vi "Save image to Tiff stack file.vi"(6 "error in":errorcluster, 8 "Tiff string\n (unsigned byte array)":u8[](array[numeric]), 9 "Path":path) -> (0 "error out":errorcluster)   [LabVIEW 2013, in "Tiff reader.lvlib"]
doc: "This .vi saves the input image to file. If the file exists, then the Tiff image is appended to the end of the file."
uses:
  Tiff reader.lvlib
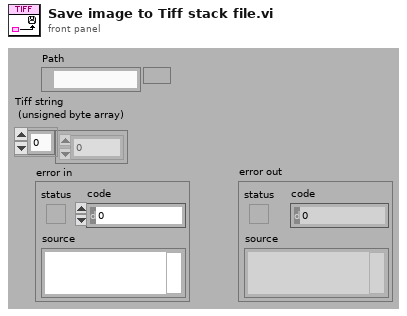
[diagram p1: front panel]
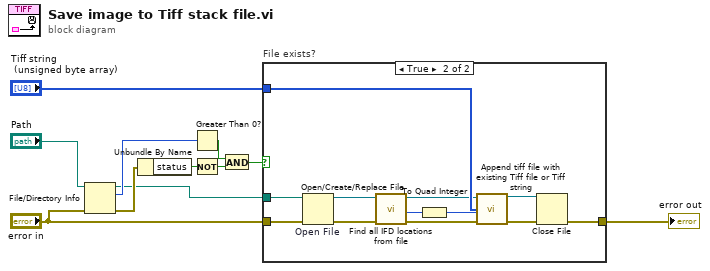
[diagram p0: block diagram]
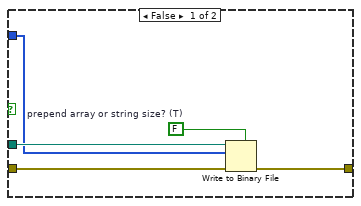
[diagram p2: hidden frame]
diagram:
  n1 = File/Directory Info(path="Path", error in="error in") -> (path out=w2:path, size=w6:i64, error out=w5:errorcluster)  [unwired: 4 out]
  n2 = Unbundle By Name(w5) -> ("status"=w7:bool)
  n3 = Greater Than 0?(x=w6) -> (x > 0?=w8:bool)
  n4 = Not(x=w7) -> (.not. x?=w9:bool)
  n5 = And(x=w8, y=w9) -> (x .and. y?=w10:bool)
  n6 = case "File exists?" shown="True" w10 {
    tunnel: [w13 w20] -> w11
    tunnel: "error in" -> [w15 w27]
    tunnel: w2 -> [w14 w28]
    tunnel: "Tiff string\n (unsigned byte array)" -> [w12 w26]
    frame False {
      w16 = FALSE  # prepend array or string size? (T)
      n7 = Write to Binary File(file (use dialog)=w14, data=w12, error in=w15, 5:w16) -> (error out=w13:errorcluster)  [unwired: 1 in, 3 out]
    }
    frame True {
      n8 = Open/Create/Replace File "Open File"(file path (use dialog)=w28, error in=w27) -> (refnum out=w25:refnum<file>, error out=w24:errorcluster)  [unwired: 5 out]
      n9 = call "Find all IFD locations from file.vi"("error in"=w24, "File"=w25) -> ("error out"=w22:errorcluster, "Location in byte stream of\n Long Word that points to the last IFD.\n\nThis is the Word to change if you are adding another page\nto the file."=w18:u32, "File"=w23:refnum<file>)  [unwired: 7 out]
      n10 = To Quad Integer(1:w18) -> (0:w17:i64)
      n11 = call "Append tiff file with existing Tiff file or Tiff string.vi"("Existing Tiff File (A) refnum"=w23, "Tiff file (B)\n (unsigned byte array)"=w26, "Location in existing file of\nit's last page's \n\"next IFD pointer\""=w17, "error in"=w22) -> ("File refnum out"=w19:refnum<file>, "error out"=w21:errorcluster)  [unwired: 3 in, 7 out]
      n12 = Close File(refnum=w19, error in=w21) -> (error out=w20:errorcluster)  [unwired: 1 out]
    }
  }
  "error out" <- w11
